vi "Analog Output (Host).vi"() -> ()   [LabVIEW 2016]
uses:
  <vilib>/FPGAPlugInAG/PXIe-7847R/niLvFpga_Open_PXIe-7847R.vi
  <vilib>/rvi/interface/common/dynamic/niFpgaDynamicAddResources.vi
  <vilib>/Utility/error.llb/Error Cluster From Error Code.vi
  <vilib>/rvi/errors/niLvFpgaAdjustHostInterfaceError.vi
  <vilib>/rvi/interface/nirviOpenFPGA/nirviOpenFPGA.xnode
  Program Files (x86)/National Instruments/LabVIEW 2016/examples/R Series/Basic IO/Analog Output/FPGA Bitfiles/AnalogOutput-test-FPGA.lvbitx
  Program Files (x86)/National Instruments/LabVIEW 2016/examples/R Series/Basic IO/Analog Output/Analog Output.vi
  <vilib>/rvi/interface/nirviReadWriteControl/nirviReadWriteControl.xnode
  NiFpgaLv.dll
  <vilib>/rvi/interface/Simulation/niFpgaSimulationCallBeginRW.vi
panel:
  in  "stop":bool
  out "Waveform Chart":dbl(graph)
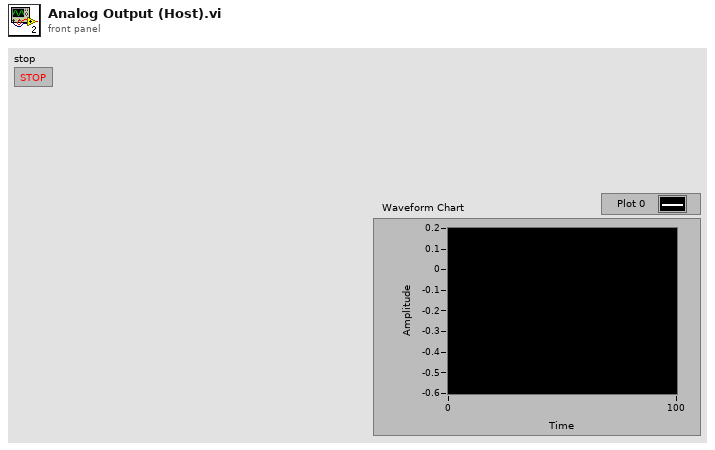
[diagram p1: front panel]
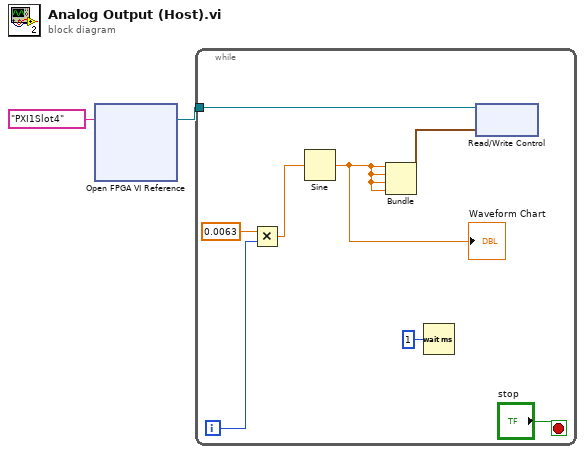
[diagram p0: block diagram]
diagram:
  n1 = xnode "Open FPGA VI Reference"("resource name"=tag "PXI1Slot4") -> ("FPGA VI Reference Out"=w2:refnum<k20>)  [unwired: 1 in, 1 out]
  n2 = while {
    tunnel: w2 -> [w10]
    i -> [w5]
    stop <- "stop" stop-if-true
    n3 = Multiply(x=0.0063, y=w5) -> (x*y=w9:dbl)
    n4 = Sine(x=w9) -> (sin(x)=w4:dbl)
    "Waveform Chart" <- w4
    n5 = Bundle(w4, w4, w4, w4) -> (w7:cluster{dbl, dbl, dbl, dbl})  [unwired: 1 in]
    n6 = Wait (ms)(milliseconds to wait=u32 1) -> ()  [unwired: 1 out]
    n7 = xnode "Read/Write Control"("FPGA VI Reference In"=w10, "AO Data"=w7) -> ()  [unwired: 1 in, 2 out]
  }
